vi "flow_strings.vi"(0 "string in":string, 1 "is first in?":bool, 2 "use source?":bool, 3 "name":string, 4 "run source?":bool, 5 "prep source?":bool, 6 "is prep?":bool) -> (7 "string out":string, 8 "is first out?":bool)   [LabVIEW 2011]
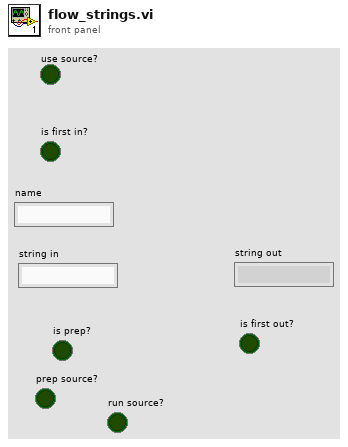
[diagram p1: front panel]
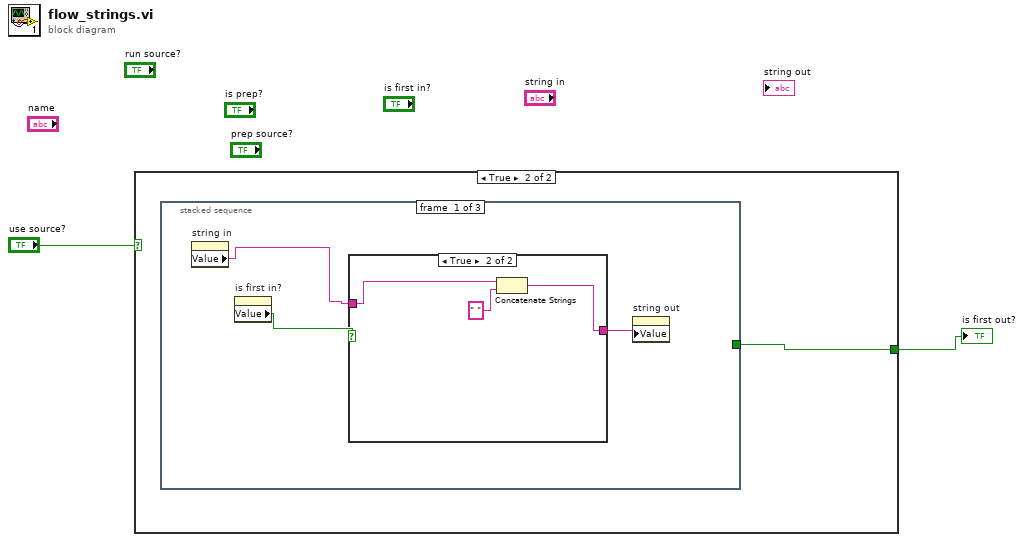
[diagram p0: block diagram]
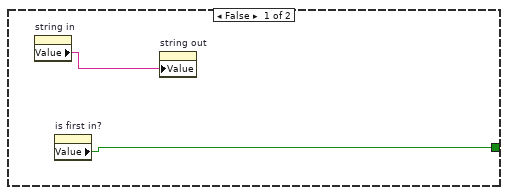
[diagram p2: hidden frame]
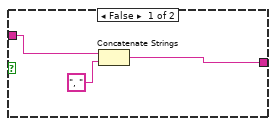
[diagram p3: hidden frame]
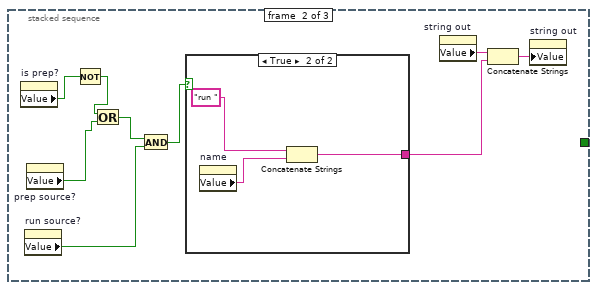
[diagram p4: hidden frame]
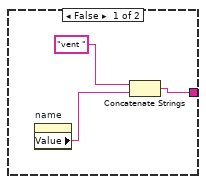
[diagram p5: hidden frame]
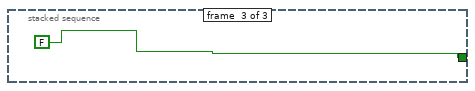
[diagram p6: hidden frame]
diagram:
  n1 = case shown="True" "use source?" {
    tunnel: [w4 w5] -> w1
    frame False {
      n2 = property on="string in" class="Str"() -> ("Value"=w3:string)  [unwired: 2 in, 2 out]
      n3 = property on="is first in?" class="Bool (strict)"() -> ("Value"=w4:bool)  [unwired: 2 in, 2 out]
      n4 = property on="string out" class="Str"("Value"=w3) -> ()  [unwired: 2 in, 2 out]
    }
    frame True {
      n5 = stacked-sequence {
        tunnel: [_ _ FALSE ("first")] -> w5
        frame #0 {
          n6 = property on="string in" class="Str"() -> ("Value"=w7:string)  [unwired: 2 in, 2 out]
          n7 = property on="is first in?" class="Bool (strict)"() -> ("Value"=w8:bool)  [unwired: 2 in, 2 out]
          n8 = case shown="True" w8 {
            tunnel: w7 -> [w11 w13]
            tunnel: [w9 w12] -> w6
            frame False {
              n9 = Concatenate Strings(w11, ", " ("string")) -> (w9:string)
            }
            frame True {
              n10 = Concatenate Strings(w13, " " ("string")) -> (w12:string)
            }
          }
          n11 = property on="string out" class="Str"("Value"=w6) -> ()  [unwired: 2 in, 2 out]
        }
        frame #1 {
          n12 = property on="is prep?" class="Bool (strict)"() -> ("Value"=w20:bool)  [unwired: 2 in, 2 out]
          n13 = property on="run source?" class="Bool (strict)"() -> ("Value"=w17:bool)  [unwired: 2 in, 2 out]
          n14 = property on="prep source?" class="Bool (strict)"() -> ("Value"=w18:bool)  [unwired: 2 in, 2 out]
          n15 = Not(x=w20) -> (.not. x?=w19:bool)
          n16 = Or(x=w19, y=w18) -> (x .or. y?=w16:bool)
          n17 = And(x=w16, y=w17) -> (x .and. y?=w15:bool)
          n18 = case shown="True" w15 {
            tunnel: [w24 w27] -> w23
            frame False {
              n19 = property on="name" class="Str"() -> ("Value"=w26:string)  [unwired: 2 in, 2 out]
              n20 = Concatenate Strings("vent ", w26) -> (w24:string)
            }
            frame True {
              n21 = property on="name" class="Str"() -> ("Value"=w28:string)  [unwired: 2 in, 2 out]
              n22 = Concatenate Strings("run ", w28) -> (w27:string)
            }
          }
          n23 = property on="string out" class="Str"() -> ("Value"=w21:string)  [unwired: 2 in, 2 out]
          n24 = Concatenate Strings(w21, w23) -> (w22:string)
          n25 = property on="string out" class="Str"("Value"=w22) -> ()  [unwired: 2 in, 2 out]
        }
        frame #2 {
        }
      }
    }
  }
  "is first out?" <- w1
